vi "GetTagsStringsAndValues.vi"() -> (3 "Strings And Values []":cluster{"String":string, "Value":u32}[](array[cluster]))   [LabVIEW 2010]
uses:
  _lib/PDLM/pdlm_lib_x86_x64_UIThread.llb/PDLM_Tag.ctl
panel:
  in  "Tag":T1 format="%x" items=["NONE"=0, "Locked"=16, "SoftLock"=17, "KeyLock"=18, "Class_IV_Lock"=20, "Interlock"=24, "LaserMode"=32, "LDH_PulsePowerTable"=33, "TriggerMode"=48, "TriggerLevelRaw"=64, "TriggerLevelRawLoLimit"=65, "TriggerLevelRawHiLimit"=66, "TriggerLevel"=72, "TriggerLevelLoLimit"=73, "TriggerLevelHiLimit"=74, "FastGate"=80, "FastGateImp"=96, "SlowGate"=112, "TargetTempRaw"=144, "TargetTempRawLoLimit"=145, "TargetTempRawHiLimit"=146, "CurrentTempRaw"=148, "CaseTempRaw"=149, "TargetTemp"=152, "TargetTempLoLimit"=153, "TargetTempHiLimit"=154, "CurrentTemp"=156, "CaseTemp"=157, "TempScale"=159, "Frequency"=168, "FrequencyLoLimit"=169, "FrequencyHiLimit"=170, "PulsePowerRaw"=176, "PulsePowerRawLoLimit"=177, "PulsePowerRawHiLimit"=178, "PulsePowerPermille"=180, "PulseShape"=181, "PulsePower"=184, "PulsePowerLoLimit"=185, "PulsePowerHiLimit"=186, "PulsePowerNanowatt"=188, "PulsePowerVoltage"=190, "PulseEnergy"=191, "CwPowerRaw"=192, "CwPowerRawLoLimit"=193, "CwPowerRawHiLimit"=194, "CwPowerPermille"=196, "CwPower"=200, "CwPowerLoLimit"=201, "CwPowerHiLimit"=202, "CwPowerMicroWatt"=204, "BurstLen"=208, "BurstPeriod"=224, "LDH_Fan"=240, "UI_Exclusive"=256]
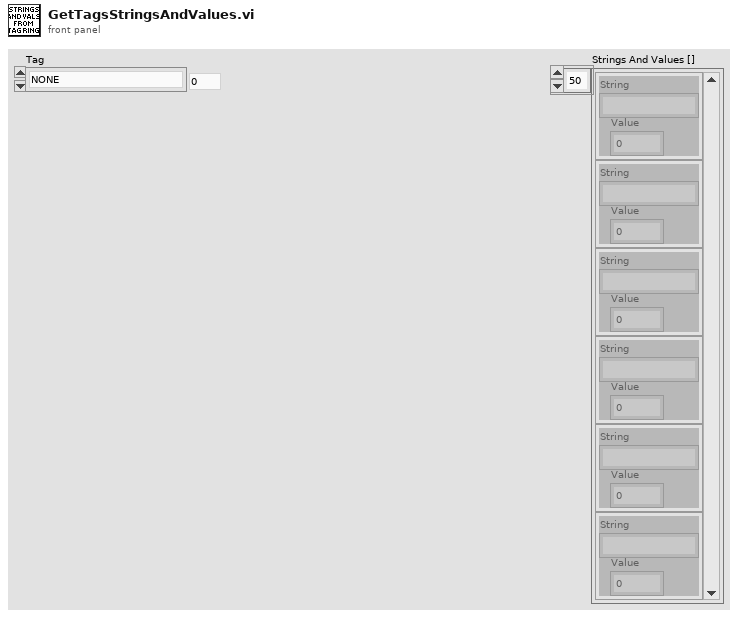
[diagram p1: front panel]
types:
  T1 = typedef "PDLM_Tag.ctl" = u32
  T2 = typedef "LVStringsAndValuesArrayTypeDef_U32.ctl" = cluster{"String":string, "Value":u32}[]
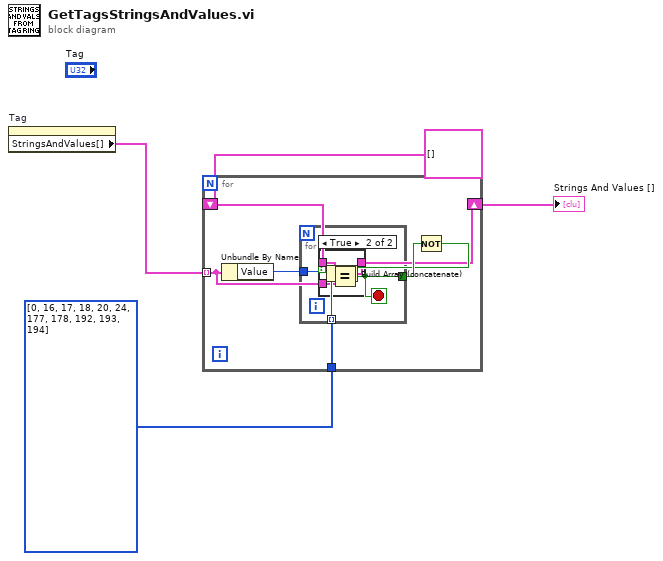
[diagram p0: block diagram]
diagram:
  n1 = property on="Tag" class="Ring (strict)"() -> ("StringsAndValues[]"=w4:T2)  [unwired: 2 in, 2 out]
  n2 = for {
    tunnel: w4 -> [w9] mode=indexing
    tunnel: u32[] [0, 16, 17, 18, 20, 24, 177, 178, 192, 193, 194] -> [w10]
    shift-right: [w5] -> w2
    shift-left: cluster{"String":string, "Value":u32}[] [] ("Array") -> [w6]
    n3 = Unbundle By Name(w9) -> ("Value"=w11:u32)
    n4 = for {
      tunnel: w11 -> [w17]
      tunnel: w10 -> [w18] mode=indexing
      tunnel: [w16] -> w8
      stop <- w16 stop-if-true
      n5 = Equal?(x=w17, y=w18) -> (x = y?=w16:bool)
    }
    n6 = Not(x=w8) -> (.not. x?=w7:bool)
    n7 = case shown="True" w7 {
      tunnel: w6 -> [w12 w14]
      tunnel: w9 -> [_ w13]
      tunnel: [w12 w15] -> w5
      frame False {
      }
      frame True {
        n8 = Build Array (concatenate)(w14, w13) -> (w15:cluster{"String":string, "Value":u32}[])
      }
    }
  }
  "Strings And Values []" <- w2
